vi "AlazarEngine.vi"(4 "Acq Settings":T1={"Window Type"=1, "Record Length"=1536, "Footer"=0, "Output Format"=11, "Offset"=0, "Records Per Buffer"=1000, "Records Count (Records/Acq)"=2147483647} {"Window Type" items=["DSP_WINDOW_NONE", "DSP_WINDOW_HANNING", "DSP_WINDOW_HAMMING", "DSP_WINDOW_BLACKMAN", "DSP_WINDOW_BLACKMAN_HARRIS", "DSP_WINDOW_BARTLETT"]; "Footer" items=["FOOTER_NONE", "FOOTER_NPT"]; "Output Format" items=["FLOAT_AMP2"=10, "FLOAT_LOG"=11]}, 6 "Trigger Settings":T8={"General Trigger Settings"={"Trigger Operation"=0, "Coupling ID"=2, "Range ID"=0, "Delay"=0, "Timeout Ticks"=0, "Mode"=0, "Parameter"=0}, "Trigger Engine 1"={"Trigger Engine"=0, "Source"=0, "Slope"=1, "Level"=0}, "Trigger Engine 2"={"Trigger Engine"=0, "Source"=0, "Slope"=1, "Level"=0}} {"General Trigger Settings"."Trigger Operation" items=["J", "K", "J OR K", "J AND K", "J XOR K", "J AND NOT K", "NOT J AND K"]; "General Trigger Settings"."Coupling ID" items=["AC"=1, "DC"=2]; "General Trigger Settings"."Range ID" items=["5 V", "1 V", "TTL"]; "Trigger Engine 1"."Trigger Engine" items=["J", "K"]; "Trigger Engine 1"."Source" items=["A", "B", "External", "Disable", "C", "D"]; "Trigger Engine 1"."Slope" items=["Positive"=1, "Negative"=2]; "Trigger Engine 2"."Trigger Engine" items=["J", "K"]; "Trigger Engine 2"."Source" items=["A", "B", "External", "Disable", "C", "D"]; "Trigger Engine 2"."Slope" items=["Positive"=1, "Negative"=2]}, 7 "Action":T2=enum."Config Trig", 8 "error in (no error)":errorcluster, 9 "Ch Input Control":T5={"Channel"=1, "Coupling"=2, "Range"=10, "Impedance"=2} {"Channel" items=["A"=1, "B"=2, "C"=4, "D"=8]; "Coupling" items=["AC"=1, "DC"=2]; "Range" items=["20 mV"=1, "40 mV"=2, "50 mV"=3, "80 mV"=4, "100 mV"=5, "200 mV"=6, "400 mV"=7, "500 mV"=8, "800 mV"=9, "1 V"=10, "1.25 V"=33, "2 V"=11, "4 V"=12, "5 V"=13, "8 V"=14, "10 V"=15, "20 V"=16]; "Impedance" items=["1 MOhm"=1, "50 Ohm"=2, ""=0]}, 10 "Capture Clock":T3={"Sample Rate"=30, "Decimation"=0, "Source"=1, "Edge"=0} {"Edge" items=["Rising", "Falling"]; "Source" items=["Internal"=1, "Fast External"=2, "Medium External"=3, "Slow External"=4, "External AC"=5, "External DC"=6, "External 10MHz"=7]}, 11 "Device ID":T4={"System ID"=1, "Board ID"=1}) -> (0 "error out":errorcluster, 2 "dt":dbl)   [LabVIEW 2018]
uses:
  Controls/General Trigger Settings.ctl
  Controls/Trigger Engine Controls.ctl
  Controls/Channel Input Controls.ctl
  Controls/Alazar Device ID.ctl
  Controls/Clock Controls.ctl
  Controls/Alazar Engine Actions.ctl
  Controls/Alazar Acquisition Settings.ctl
  Controls/Async Read Parameters.ctl
  General/Controls/FGV Actions.ctl
  General/Queue Manager Actions.ctl
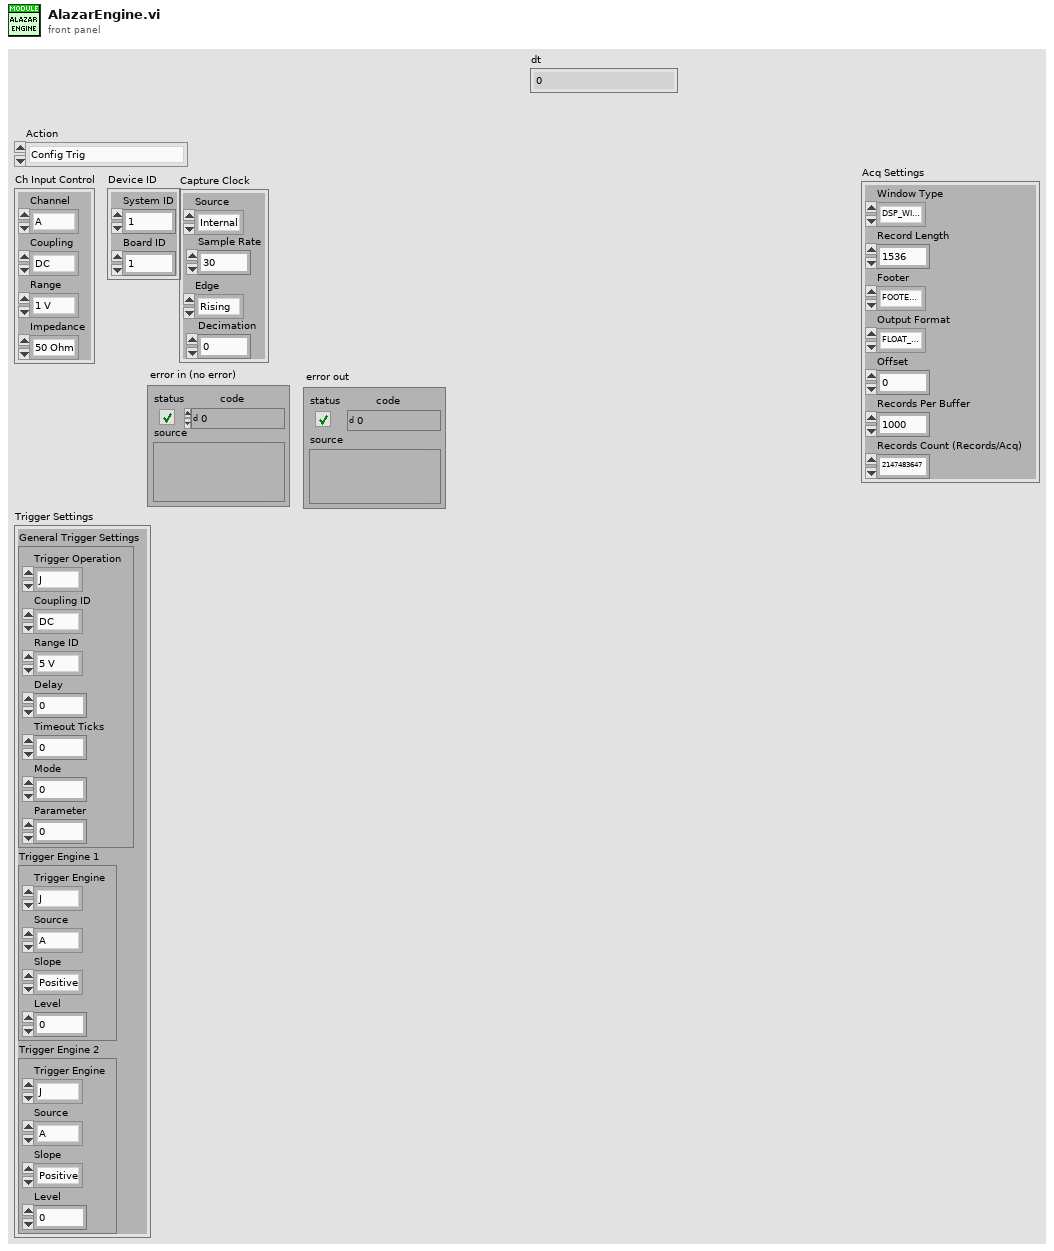
[diagram p1: front panel]
types:
  T1 = typedef "Alazar Acquisition Settings.ctl" = cluster{"Window Type":u32, "Record Length":u32, "Footer":u32, "Output Format":u32, "Offset":u32, "Records Per Buffer":u32, "Records Count (Records/Acq)":u32}
  T2 = typedef "Alazar Engine Actions.ctl" = enum16{"Init", "Config Clock", "Config Ch", "Config Trig", "Config Acq.", "Acquire", "UnInit"}
  T3 = typedef "Clock Controls.ctl" = cluster{"Sample Rate":u32, "Decimation":u32, "Source":u32, "Edge":u32}
  T4 = typedef "Alazar Device ID.ctl" = cluster{"System ID":u32, "Board ID":u32}
  T5 = typedef "Channel Input Controls.ctl" = cluster{"Channel":u8, "Coupling":u32, "Range":u32, "Impedance":u32}
  T6 = typedef "General Trigger Settings.ctl" = cluster{"Trigger Operation":u32, "Coupling ID":u32, "Range ID":u32, "Delay":u32, "Timeout Ticks":u32, "Mode":u32, "Parameter":u32}
  T7 = typedef "Trigger Engine Controls.ctl" = cluster{"Trigger Engine":u32, "Source":u32, "Slope":u32, "Level":u32}
  T8 = cluster{"General Trigger Settings":T6, "Trigger Engine 1":T7, "Trigger Engine 2":T7}
  T9 = typedef "FGV Actions.ctl" = enum16{"Init", "Set", "Get", "Clear"}
  T10 = typedef "Async Read Parameters.ctl" = cluster{"Transfer Offset":u32, "Transfer Length":u32, "Records Per Buffer":u32, "Records Per Acquisition":u32}
  T11 = typedef "Queue Manager Actions.ctl" = enum16{"Init", "Enqueue", "Enqueue All", "Preview Queue", "Dequeue", "Get Status", "Flush Queue", "Flush All Queues", "Release All Queues", "Release Queue", "Enqueue at Opposite End"}
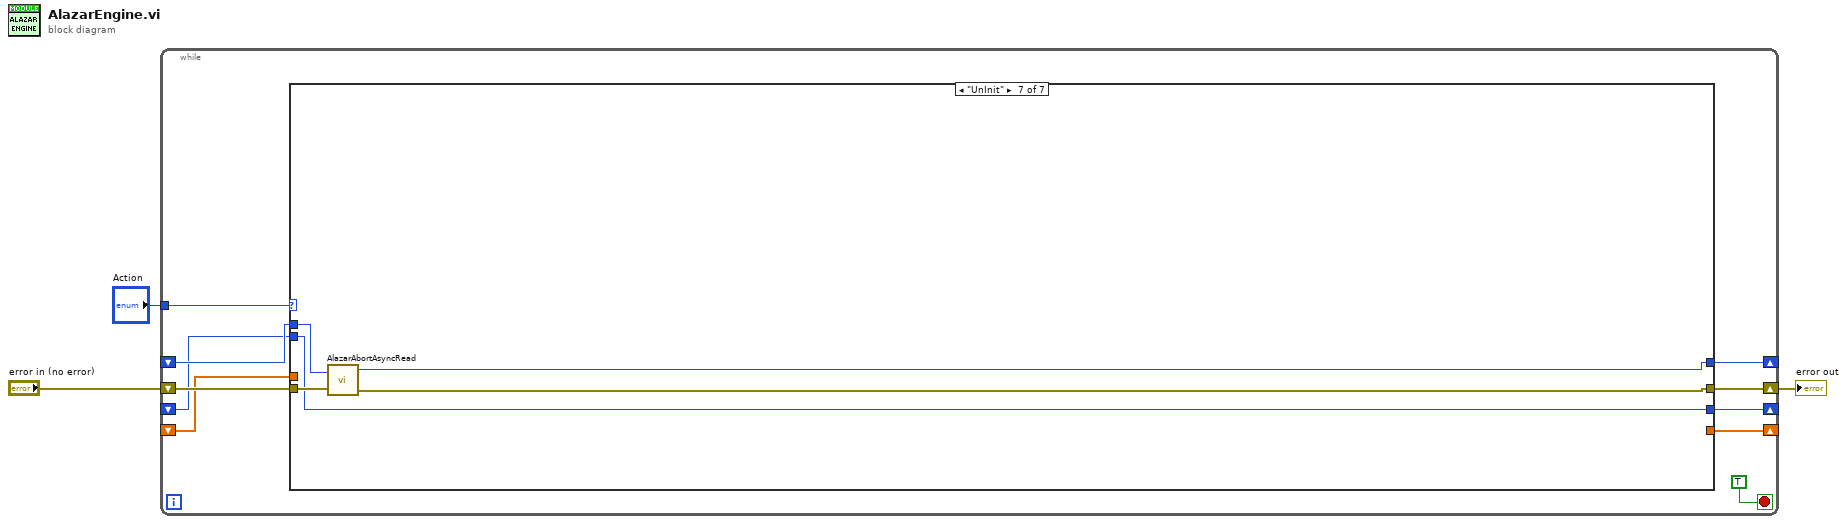
[diagram p0: block diagram]
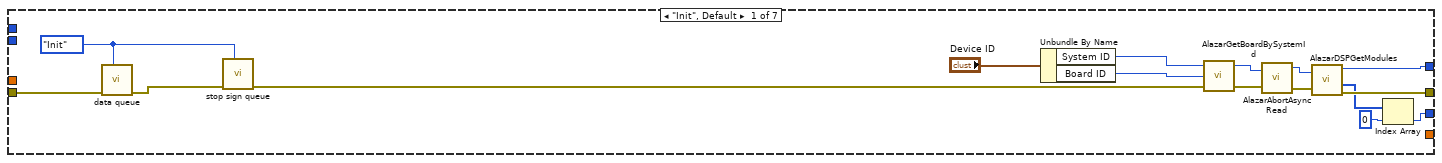
[diagram p2: hidden frame]
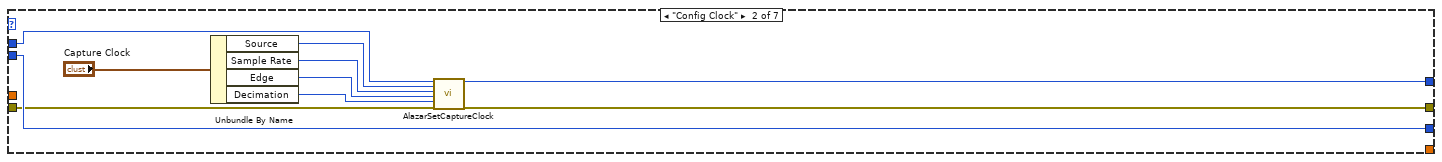
[diagram p3: hidden frame]
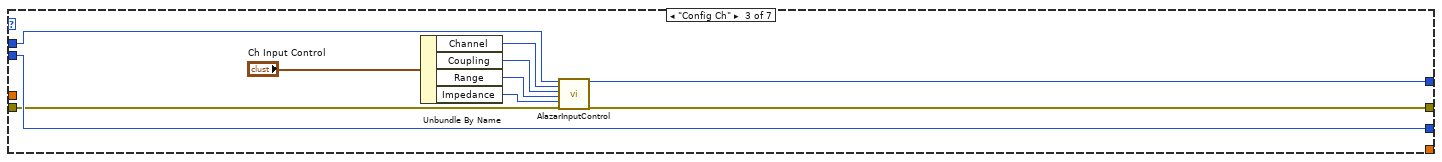
[diagram p4: hidden frame]
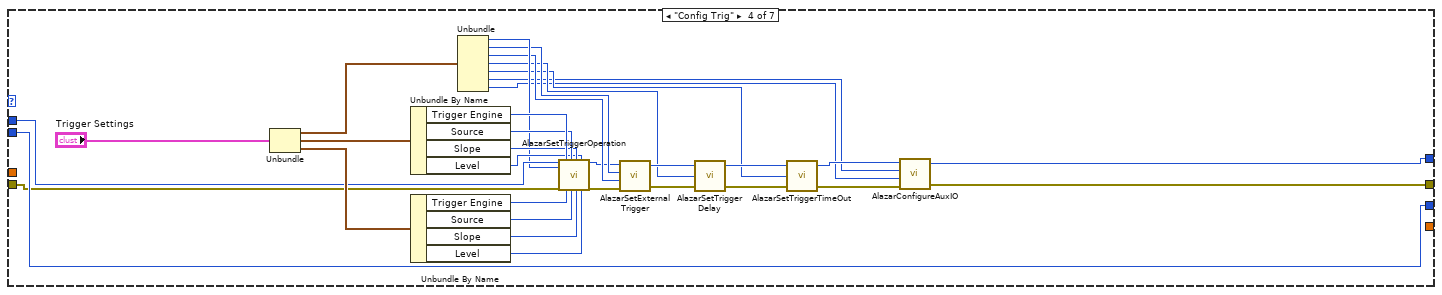
[diagram p5: hidden frame]
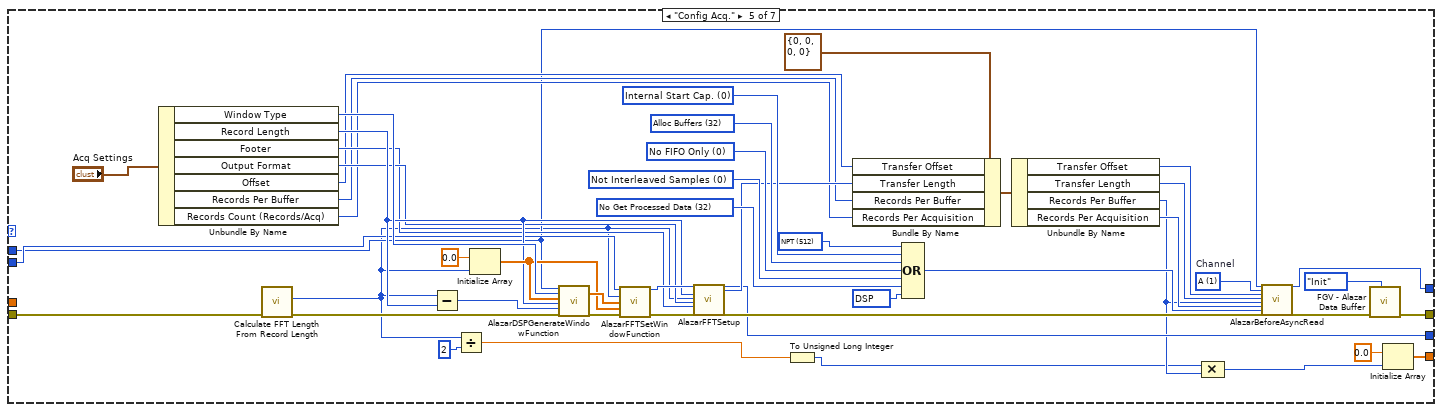
[diagram p6: hidden frame]
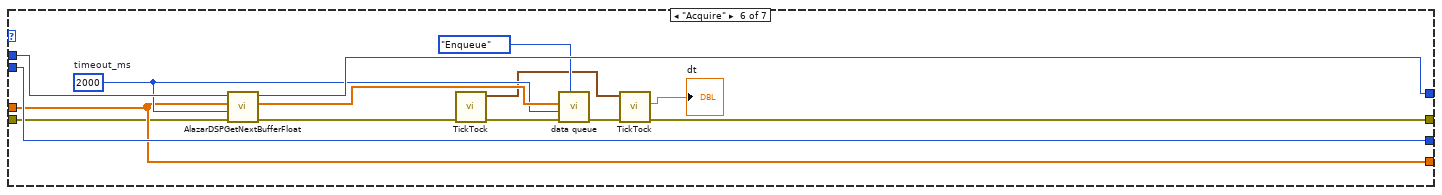
[diagram p7: hidden frame]
diagram:
  n1 = while {
    tunnel: "Action" -> [w11]
    shift-right: [w10] -> _
    shift-left: _ -> [w9]
    shift-right: [w8] -> _
    shift-left: _ -> [w7]
    shift-right: [w6] -> w1
    shift-left: "error in (no error)" -> [w12]
    shift-right: [w5] -> _
    shift-left: _ -> [w4]
    stop <- TRUE stop-if-true
    n2 = case shown="\"UnInit\"" w11 {
      tunnel: w12 -> [w17 w37 w43 w63 w119 w131 w147]
      tunnel: [w20 w30 w42 w51 w120 w135 w148] -> w6
      tunnel: [w18 w31 w41 w50 w92 w142 w145] -> w10
      tunnel: w9 -> [_ w32 w40 w68 w99 w143 w146]
      tunnel: [w28 w39 w49 w79 w90 w141 w144] -> w8
      tunnel: w7 -> [_ w39 w49 w79 w106 w141 w144]
      tunnel: [_ _ _ _ w83 w137 _] -> w5
      tunnel: w4 -> [_ _ _ _ _ w137 _]
      frame "Init", Default {
        w14 = Queue_Manager_Actions."Init" ("Action")
        n3 = call "data queue.vi"("Action"=w14, "error in (no error)"=w17) -> ("error out"=w16:errorcluster)  [unwired: 6 in, 3 out]
        n4 = call "stop sign queue.vi"("Action"=w14, "error in (no error)"=w16) -> ("error out"=w15:errorcluster)  [unwired: 6 in, 3 out]
        n5 = Unbundle By Name("Device ID") -> ("System ID"=w26:u32, "Board ID"=w25:u32)
        n6 = call "AlazarGetBoardBySystemId.vi"("error in (no error)"=w15, "Board ID"=w25, "System ID"=w26) -> ("error out"=w24:errorcluster, "Handle"=w23:u64)  [unwired: 1 out]
        n7 = call "AlazarAbortAsyncRead.vi"("Handle"=w23, "error in (no error)"=w24) -> ("Handle"=w22:u64, "error out"=w21:errorcluster)  [unwired: 1 out]
        n8 = call "AlazarDSPGetModules.vi"("Handle"=w22, "error in (no error)"=w21) -> ("Handle"=w18:u64, "DSP Modules"=w19:u64[], "error out"=w20:errorcluster)  [unwired: 1 out]
        n9 = Index Array(array=w19, index=u32 0) -> (element=w28:u64)
      }
      frame "Config Clock" {
        n10 = Unbundle By Name("Capture Clock") -> ("Source"=w33:u32, "Sample Rate"=w34:u32, "Edge"=w35:u32, "Decimation"=w36:u32)
        n11 = call "AlazarSetCaptureClock.vi"("Handle"=w32, "Source"=w33, "Sample Rate"=w34, "Edge"=w35, "Decimation"=w36, "error in (no error)"=w37) -> ("Handle"=w31:u64, "error out"=w30:errorcluster)  [unwired: 11 in, 1 out]
      }
      frame "Config Ch" {
        n12 = Unbundle By Name("Ch Input Control") -> ("Channel"=w47:u8, "Coupling"=w46:u32, "Range"=w45:u32, "Impedance"=w44:u32)
        n13 = call "AlazarInputControl.vi"("Handle"=w40, "Channel"=w47, "Coupling"=w46, "Range"=w45, "Impedance"=w44, "error in (no error)"=w43) -> ("Handle"=w41:u64, "error out"=w42:errorcluster)  [unwired: 11 in, 1 out]
      }
      frame "Config Trig" {
        n14 = Unbundle("Trigger Settings") -> ("General Trigger Settings"=w80:T6, "Trigger Engine 1"=w78:T7, "Trigger Engine 2"=w77:T7)
        n15 = Unbundle By Name(w78) -> ("Trigger Engine"=w76:u32, "Source"=w75:u32, "Slope"=w74:u32, "Level"=w73:u32)
        n16 = Unbundle By Name(w77) -> ("Trigger Engine"=w72:u32, "Source"=w71:u32, "Slope"=w70:u32, "Level"=w69:u32)
        n17 = Unbundle(w80) -> ("Trigger Operation"=w67:u32, "Coupling ID"=w66:u32, "Range ID"=w65:u32, "Delay"=w59:u32, "Timeout Ticks"=w56:u32, "Mode"=w53:u32, "Parameter"=w52:u32)
        n18 = call "AlazarSetTriggerOperation.vi"("Handle"=w68, "Trigger Operation"=w67, "error in (no error)"=w63, "Trigger Engine 1"=w76, "Trigger Engine 2"=w72, "Source 1"=w75, "Source 2"=w71, "Slope 1"=w74, "Slope 2"=w70, "Level 1"=w73, "Level 2"=w69) -> ("Handle"=w61:u64, "error out"=w64:errorcluster)  [unwired: 6 in, 1 out]
        n19 = call "AlazarSetExternalTrigger.vi"("error in (no error)"=w64, "Range ID"=w65, "Coupling ID"=w66, "Handle"=w61) -> ("error out"=w62:errorcluster, "Handle"=w60:u64)  [unwired: 1 out]
        n20 = call "AlazarSetTriggerDelay.vi"("error in (no error)"=w62, "Delay"=w59, "Handle"=w60) -> ("error out"=w58:errorcluster, "Handle"=w57:u64)  [unwired: 1 out]
        n21 = call "AlazarSetTriggerTimeOut.vi"("error in (no error)"=w58, "Timeout Ticks"=w56, "Handle"=w57) -> ("error out"=w55:errorcluster, "Handle"=w54:u64)  [unwired: 1 out]
        n22 = call "AlazarConfigureAuxIO.vi"("error in (no error)"=w55, "Parameter"=w52, "Mode"=w53, "Handle"=w54) -> ("error out"=w51:errorcluster, "Handle"=w50:u64)  [unwired: 1 out]
      }
      frame "Config Acq." {
        w122 = u32 16384 items=["DSP"=16384]
        w98 = u32 1 items=["A"=1]  # Channel
        w128 = u32 32 items=["No Get Processed Data"=32, "Get Processed Data"=8192]
        w127 = u32 0 items=["Not Interleaved Samples"=0, "Interleave Samples"=4096]
        w123 = u32 0 items=["No FIFO Only"=0, "FIFO Only"=2048]
        w126 = u32 32 items=["Alloc Buffers"=32]
        w125 = u32 0 items=["Internal Start Cap.", "External Start Cap."]
        w124 = u32 512 items=["Traditional"=0, "NPT"=512, "Continuous"=256, "Triggered Streaming"=1024]
        n23 = Unbundle By Name("Acq Settings") -> ("Window Type"=w116:u32, "Record Length"=w110:u32, "Footer"=w108:u32, "Output Format"=w109:u32, "Offset"=w104:u32, "Records Per Buffer"=w102:u32, "Records Count (Records/Acq)"=w101:u32)
        n24 = call "Calculate FFT Length From Record Length.vi"("error in (no error)"=w119) -> ("error out"=w117:errorcluster, "FFT Length"=w88:u32)  [unwired: 8 in, 1 out]
        n25 = Subtract(x=w88, y=w110) -> (x-y=w115:u32)
        n26 = Divide(x=w88, y=u32 2) -> (x/y=w84:dbl)
        n27 = Initialize Array(sgl 0.0, w88) -> (w113:sgl[])
        n28 = call "AlazarDSPGenerateWindowFunction.vi"("Handle"=w99, "Window Type"=w116, "window"=w113, "WindowLength_samples"=w110, "PaddingLength_samples"=w115, "error in (no error)"=w117) -> ("window"=w114:sgl[], "error out"=w112:errorcluster)  [unwired: 10 in, 2 out]
        n29 = call "AlazarFFTSetWindowFunction.vi"("DSP Handle"=w106, "Samples per record"=w88, "Real window array"=w114, "Imag window array"=w113, "error in (no error)"=w112) -> ("DSP Handle"=w111:u64, "error out"=w107:errorcluster)  [unwired: 9 in]
        n30 = call "AlazarFFTSetup.vi"("DSP Handle"=w111, "Record Length (samples)"=w110, "FFT Length (samples)"=w88, "Output Format"=w109, "Footer"=w108, "error in (no error)"=w107) -> ("DSP Handle"=w90:u64, "Bytes Per Output Record"=w103:u32, "error out"=w91:errorcluster)  [unwired: 18 in, 1 out]
        n31 = To Unsigned Long Integer(number=w84) -> (unsigned 32bit integer=w82:u32)
        n32 = Bundle By Name(cluster=T10 {"Transfer Offset"=0, "Transfer Length"=0, "Records Per Buffer"=0, "Records Per Acquisition"=0} ("ASync Read Parameters"), "Transfer Offset"=w104, "Transfer Length"=w103, "Records Per Buffer"=w102, "Records Per Acquisition"=w101) -> (w100:T10)
        n33 = Compound Arithmetic op=OR(w124, w125, w126, w123, w127, w128, w122) -> (w94:u32)
        n34 = Unbundle By Name(w100) -> ("Transfer Offset"=w97:u32, "Transfer Length"=w96:u32, "Records Per Buffer"=w89:u32, "Records Per Acquisition"=w95:u32)
        n35 = Compound Arithmetic op=MULTIPLY(w82, w89) -> (w87:u32)
        n36 = call "AlazarBeforeAsyncRead.vi"("Handle"=w99, "Channel Select"=w98, "Transfer Offset"=w97, "Transfer Length"=w96, "Records Per Buffer"=w89, "Records Per Acquisition"=w95, "Flags"=w94, "error in (no error)"=w91) -> ("Handle"=w92:u64, "error out"=w93:errorcluster)  [unwired: 17 in, 1 out]
        n37 = call "FGV - Alazar Data Buffer.vi"("Actions"=FGV_Actions."Init", "error in (no error)"=w93) -> ("error out"=w120:errorcluster)  [unwired: 8 in, 1 out]
        n38 = Initialize Array(0.0 ("element"), w87) -> (w83:dbl[])
      }
      frame "Acquire" {
        w138 = u32 2000  # timeout_ms
        n39 = call "AlazarDSPGetNextBufferFloat.vi"("error in (no error)"=w131, "timeout_ms"=w138, "Buffer"=w137, "Handle"=w143) -> ("error out"=w130:errorcluster, "Buffer"=w140:sgl[], "Handle"=w142:u64)  [unwired: 1 out]
        n40 = call "TickTock.vi"("Error In"=w130) -> ("Error Out"=w133:errorcluster, "Current Time (Out)"=w132:timestamp)  [unwired: 8 in, 1 out]
        n41 = call "data queue.vi"("Action"=Queue_Manager_Actions."Enqueue", "error in (no error)"=w133, "timeout in ms (-1)"=w138, "data in"=w140) -> ("error out"=w136:errorcluster)  [unwired: 4 in, 3 out]
        n42 = call "TickTock.vi"("Error In"=w136, "Current Time (In)"=w132) -> ("Error Out"=w135:errorcluster, "dt"=→"dt":dbl)  [unwired: 7 in, 1 out]
      }
      frame "UnInit" {
        n43 = call "AlazarAbortAsyncRead.vi"("Handle"=w146, "error in (no error)"=w147) -> ("Handle"=w145:u64, "error out"=w148:errorcluster)  [unwired: 1 out]
      }
    }
  }
  "error out" <- w1
